vi "Initialize.vi"(4 "Log Directory":path, 6 "Resource":string, 7 "Instance Name":string, 8 "error in (no error)":errorcluster, 9 "Receiving Queue":refnum<queue>, 10 "Control Panel Path":path, 11 "Controller Type":T1) -> (0 "error out":errorcluster, 2 "Failed?":bool, 3 "Plugin Server out":refnum<class "Generic Plugin.lvclass">)   [LabVIEW 2020, in "RxnRover.lvlib" / "Generic Plugin.lvclass"]
doc: "Initializes the internals of the plugin server."
uses:
  Generic Plugin.lvclass
  Controller Type.ctl
  <userlib>/RxnRover/DynamicReentrant/src/Type Defs/Message.ctl
  Generic Plugin.lvclass/Generic Plugin.ctl
  <userlib>/RxnRover/DynamicReentrant/Dynamic Reentrant.lvlib
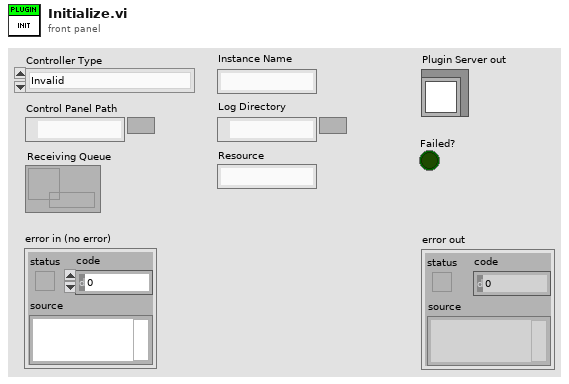
[diagram p1: front panel]
types:
  T1 = typedef "RxnRover.lvlib/Generic Plugin.lvclass/Controller Type.ctl" = enum16{"Invalid", "Temperature Controller", "Pump Controller", "Syringe Pump", "Generic Optimizer", "LC Parser"}
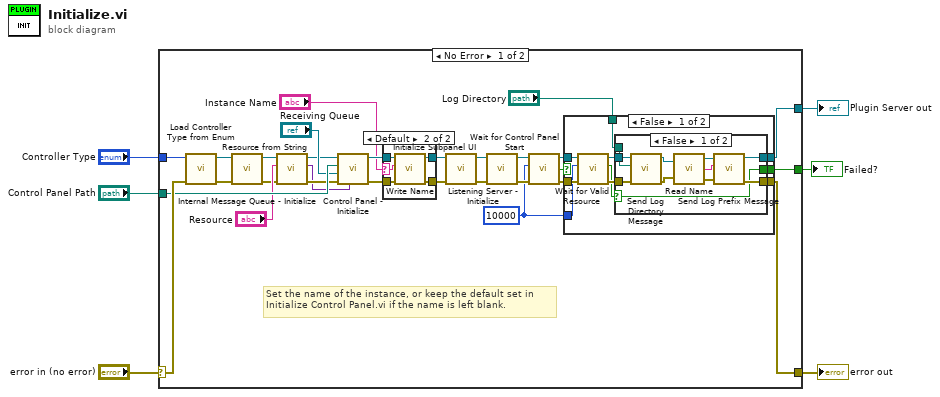
[diagram p0: block diagram]
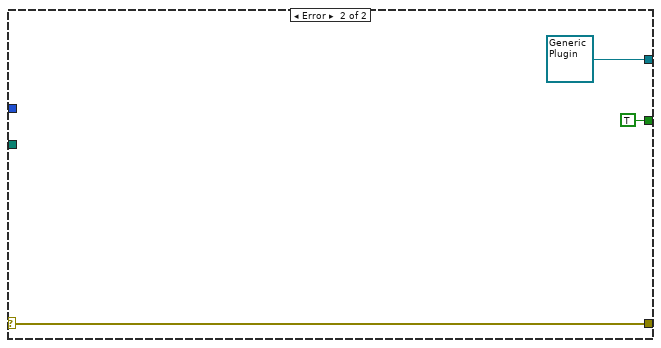
[diagram p5: hidden frame]
diagram:
  n1 = case shown="No Error" "error in (no error)" {
    selector: "error in (no error)" -> [w35 w72]
    tunnel: [w22 w72] -> w5
    tunnel: [w21 refnum<class "Generic Plugin.lvclass"> refnum ("Controller out")] -> w4
    tunnel: "Controller Type" -> [w31 _]
    tunnel: "Control Panel Path" -> [w34 _]
    tunnel: [w7 TRUE] -> w1
    frame No Error {
      w9 = 10000 ("timeout in ms (-1)")
      # "Set the name of the instance, or keep the default set in \nInitialize Control Panel.vi if the name is left blank."
      n2 = call "Load Controller Type from Enum.vi"("error in (no error)"=w35, "Controller Type"=w31) -> ("error out"=w33:errorcluster, "controller out"=w26:refnum<class "Generic Plugin.lvclass">)  [unwired: 8 in]
      n3 = call "Internal Message Queue - Initialize.vi"("error in (no error)"=w33, "Generic Controller in"=w26) -> ("error out"=w12:errorcluster, "Generic Controller out"=w15:refnum<class "Generic Plugin.lvclass">)  [unwired: 8 in]
      n4 = call-dynamic "Resource from String.vi"("error in (no error)"=w12, "Resource from String"="Resource", "Generic Controller in"=w15) -> ("error out"=w11:errorcluster, "Resource as Variant"=w10:variant, "Generic Controller out"=w14:refnum<class "Generic Plugin.lvclass">)  [unwired: 6 in]
      n5 = call "Control Panel - Initialize.vi"("Resource"=w10, "error in (no error)"=w11, "Receiving Queue"="Receiving Queue", "Control Panel Path"=w34, "Plugin Server in"=w14) -> ("error out"=w18:errorcluster, "Plugin Server out"=w30:refnum<class "Generic Plugin.lvclass">)  [unwired: 5 in]
      n6 = case shown="Default" "Instance Name" {
        selector: "Instance Name" -> [_ w65]
        tunnel: w30 -> [w64 w69]
        tunnel: [w64 w68] -> w19
        tunnel: w18 -> [w63 w67]
        tunnel: [w63 w66] -> w17
        frame "" {
        }
        frame Default {
          n7 = call "Write Name.vi"("error in (no error)"=w67, "Name"=w65, "controller in"=w69) -> ("error out"=w66:errorcluster, "controller out"=w68:refnum<class "Generic Plugin.lvclass">)  [unwired: 7 in]
        }
      }
      n8 = call "Initialize Subpanel UI.vi"("error in (no error)"=w17, "Plugin in"=w19) -> ("error out"=w32:errorcluster, "Plugin out"=w28:refnum<class "Generic Plugin.lvclass">)  [unwired: 7 in, 1 out]
      n9 = call "Listening Server - Initialize.vi"("error in (no error)"=w32, "Plugin in"=w28) -> ("error out"=w29:errorcluster, "Plugin out"=w27:refnum<class "Generic Plugin.lvclass">)  [unwired: 7 in, 1 out]
      n10 = call "Wait for Control Panel Start.vi"("error in (no error)"=w29, "timeout in ms (-1)"=w9, "Generic Controller in"=w27) -> ("error out"=w25:errorcluster, "Timeout?"=w8:bool, "Generic Controller out"=w20:refnum<class "Generic Plugin.lvclass">)  [unwired: 6 in]
      n11 = case shown="False" w8 {
        selector: w8 -> [_ w60]
        tunnel: w25 -> [w45 w61]
        tunnel: "Log Directory" -> [w44 _]
        tunnel: [w43 w61] -> w22
        tunnel: [w42 w62] -> w21
        tunnel: w20 -> [w40 w62]
        tunnel: w9 -> [w37 _]
        tunnel: [w36 w60] -> w7
        frame False {
          n12 = call "Wait for Valid Resource.vi"("error in (no error)"=w45, "timeout in ms (-1)"=w37, "Generic Controller in"=w40) -> ("error out"=w41:errorcluster, "Timeout?"=w38:bool, "Generic Controller out"=w39:refnum<class "Generic Plugin.lvclass">)  [unwired: 6 in]
          n13 = case shown="False" w38 {
            selector: w38 -> [w46 w57]
            tunnel: w44 -> [w56 _]
            tunnel: [w55 w58] -> w43
            tunnel: [w54 w59] -> w42
            tunnel: w41 -> [w48 w58]
            tunnel: w39 -> [w47 w59]
            tunnel: [w46 w57] -> w36
            frame False {
              n14 = call "Send Log Directory Message.vi"("error in (no error)"=w48, "Log Directory"=w56, "Generic Controller in"=w47) -> ("error out"=w53:errorcluster, "Generic Controller out"=w51:refnum<class "Generic Plugin.lvclass">)  [unwired: 7 in]
              n15 = call "Read Name.vi"("controller in"=w51, "error in (no error)"=w53) -> ("controller out"=w50:refnum<class "Generic Plugin.lvclass">, "Name"=w49:string, "error out"=w52:errorcluster)
              n16 = call "Send Log Prefix Message.vi"("error in (no error)"=w52, "Log Prefix"=w49, "Generic Controller in"=w50) -> ("error out"=w55:errorcluster, "Generic Controller out"=w54:refnum<class "Generic Plugin.lvclass">)  [unwired: 7 in]
            }
            frame True {
            }
          }
        }
        frame True {
        }
      }
    }
    frame Error {
    }
  }
  "error out" <- w5
  "Plugin Server out" <- w4
  "Failed?" <- w1
